vi "log_rt_error.vi"(8 "error in (no error)":errorcluster caption="错误输入（无错误）", 10 "Error Log Path":path caption="错误记录路径", 11 "Log Entry":string caption="记录输入") -> (0 "error out":errorcluster caption="错误输出")   [LabVIEW 2015]
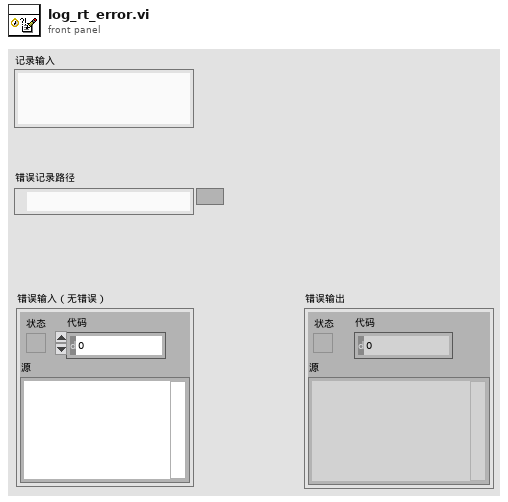
[diagram p1: front panel]
types:
  T1 = enum16{"open", "replace", "create", "open or create", "replace or create", "replace or create with confirmation"}
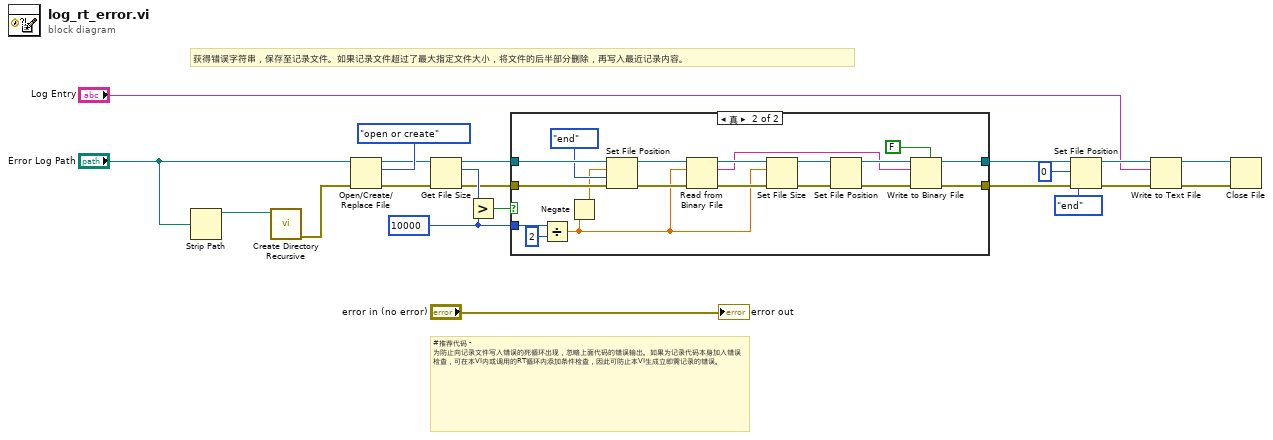
[diagram p0: block diagram]
diagram:
  w1 = i64 10000
  # "#推荐代码 - 为防止向记录文件写入错误的死循环出现，忽略上面代码的错误输出。如果为记录代码本身加入错误检查，可在本VI内或调用的RT循环内添加条件检查，因此可防止本VI生成立即需记录的错误。"
  # "获得错误字符串，保存至记录文件。如果记录文件超过了最大指定文件大小，将文件的后半部分删除，再写入最近记录内容。"
  n1 = Strip Path(path="Error Log Path") -> (stripped path=w6:path)  [unwired: 1 out]
  n2 = call <vilib>:"Create Directory Recursive.vi"("directory"=w6) -> ("error out"=w7:errorcluster)  [unwired: 4 in, 2 out]
  n3 = Open/Create/Replace File(file path (use dialog)="Error Log Path", error in=w7, operation (0:open)=T1."open or create") -> (refnum out=w8:refnum<file>, error out=w9:errorcluster)  [unwired: 2 in, 2 out]
  n4 = Get File Size(file=w8, error in=w9) -> (refnum out=w14:refnum<file>, size (in bytes)=w16:i64, 0:w13:errorcluster)
  n5 = Greater?(x=w16, y=w1) -> (0:w15:bool)
  n6 = case shown="真" w15 {
    tunnel: w14 -> [w23 w41]
    tunnel: w13 -> [w22 w42]
    tunnel: w1 -> [_ w38]
    tunnel: [w23 w26] -> w12
    tunnel: [w22 w25] -> w11
    frame False {
    }
    frame True {
      n7 = Divide(x=w38, y=i64 2) -> (x/y=w33:dbl)
      n8 = Negate(x=w33) -> (-x=w24:dbl)
      n9 = Set File Position(offset (in bytes) (0)=w24, refnum=w41, from (0:start)=enum16{"start", "end", "current"}."end", error in=w42) -> (refnum out=w36:refnum<file>, error out=w37:errorcluster)
      n10 = Read from Binary File(8:w37, 10:w33, 11:w36) -> (0:w34:errorcluster, 2:w27:string, 3:w35:refnum<file>)  [unwired: 3 in, 1 out]
      n11 = Set File Size(4:w34, 6:w33, 7:w35) -> (0:w32:errorcluster, 3:w31:refnum<file>)
      n12 = Set File Position(refnum=w31, error in=w32) -> (refnum out=w29:refnum<file>, error out=w30:errorcluster)  [unwired: 2 in]
      n13 = Write to Binary File(file (use dialog)=w29, data=w27, error in=w30, 5:FALSE ("prepend array or string size? (T)")) -> (refnum out=w26:refnum<file>, error out=w25:errorcluster)  [unwired: 2 in, 1 out]
    }
  }
  n14 = Set File Position(offset (in bytes) (0)=i64 0, refnum=w12, from (0:start)=enum16{"start", "end", "current"}."end", error in=w11) -> (refnum out=w19:refnum<file>, error out=w18:errorcluster)
  n15 = Write to Text File(file (use dialog)=w19, text="Log Entry", error in=w18) -> (refnum out=w21:refnum<file>, error out=w20:errorcluster)  [unwired: 1 in, 1 out]
  n16 = Close File(refnum=w21, error in=w20) -> ()  [unwired: 2 out]
  "error out" <- "error in (no error)"
